vi "Durability_will_2012_07_05_long filesave working.vi"() -> ()   [LabVIEW 2011]
uses:
  <vilib>/DAQmx/write.llb/DAQmx Write (Counter Time 1Chan 1Samp).vi
  <vilib>/DAQmx/read.llb/DAQmx Read (Analog 1D Wfm NChan NSamp).vi
  <vilib>/express/express shared/ex_Modify Signal Name.vi
  <vilib>/measure/madcrms.llb/Basic Averaged DC-RMS for 1 Chan.vi
  <vilib>/DAQmx/miscellaneous.llb/DAQmx Fill In Error Info.vi
  <vilib>/express/express arith-compare/Formula/XNode/ExpressFormulaBlockNode.xnode
  <vilib>/measure/NI_MAPro.lvlib
  <vilib>/Analysis/NI_AALBase.lvlib
panel:
  out "Long":bool caption="Time has Elapsed"
  out "Short":bool caption="Time has Elapsed"
  out "Temps":dynamicdata(graph) caption="Signal Out"
  in  "View Short File":bool
  in  "View Long File":bool
  out "Power Graph":dynamicdata(graph) caption="Collected Signals"
  out "Errors":errorcluster
  out "RPM":dynamicdata(graph) caption="Collected Signals"
  in  "Long Filename":path=path "C:/Users/Will/Documents/LabVIEW Data/Durability/long.tdms" caption="Filename"
  in  "Short Filename":path=path "C:/Users/Will/Documents/LabVIEW Data/Durability/short.tdms" caption="Filename"
  out "Motor RPM":dbl format="%#.0f"
  out "Motor Power (watts)":dbl format="%#.4f"
  out "Power to MC1 (watts)":dbl format="%#.4f"
  out "Voltage to MC1 (volts)":dbl format="%#.4f"
  out "Current to MC1  (amps)":dbl format="%#.4f"
  in  "Manual Start":bool
  in  "Power \nSetting":i8(slide) min=0 max=100 step=10 scale=0.0..100.0
  out "Power Setting (%)":dbl format="%#.2f"
  out "Motor Temp (F)":dbl format="%.1f"
  out "Tank Temp (F)":dbl format="%.1f"
  in  "Quit 4":bool
  out "Motor Power Over Time":dbl(graph)
  out "Phase to Phase Voltage":waveform(dbl)(graph)
  out "Phase Current":waveform(dbl)(graph)
  # "Motor Power and RPM"
  # "Temperature"
  # "MC1"
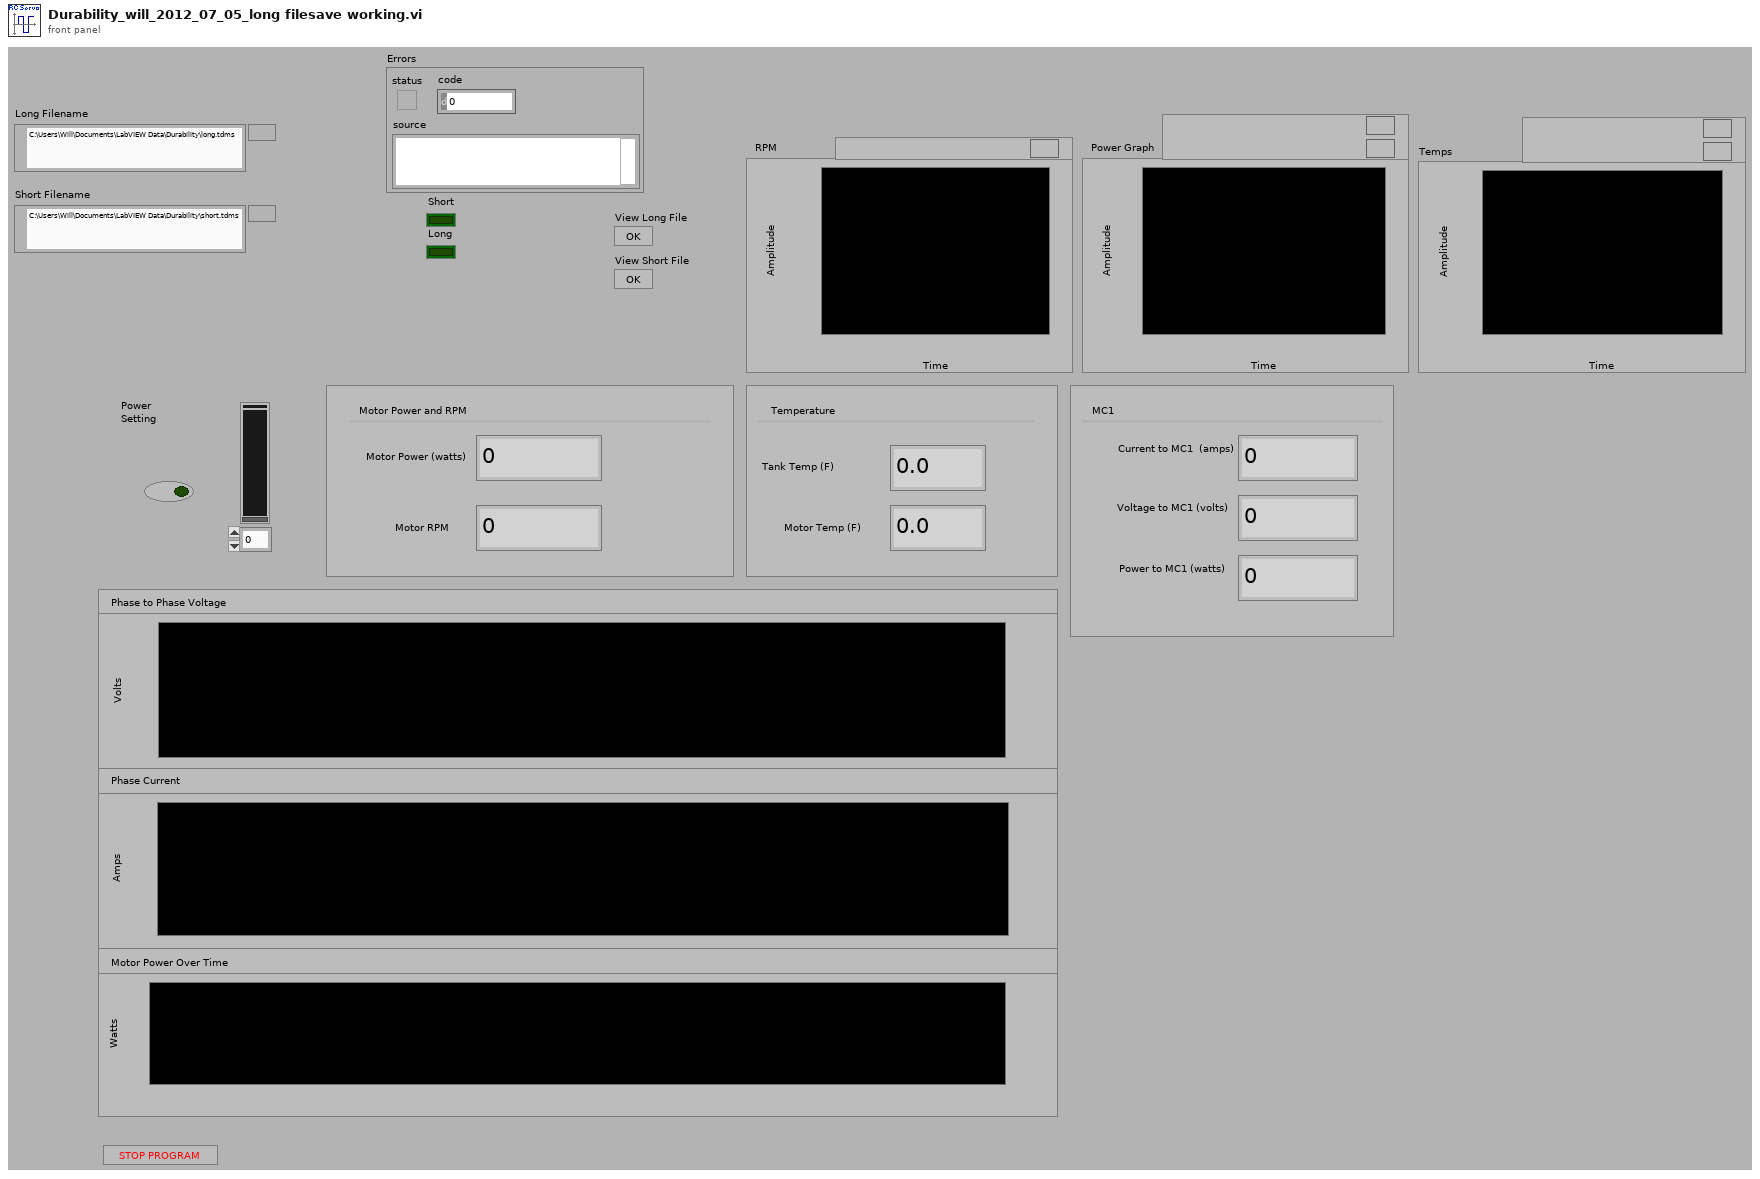
[diagram p1: front panel]
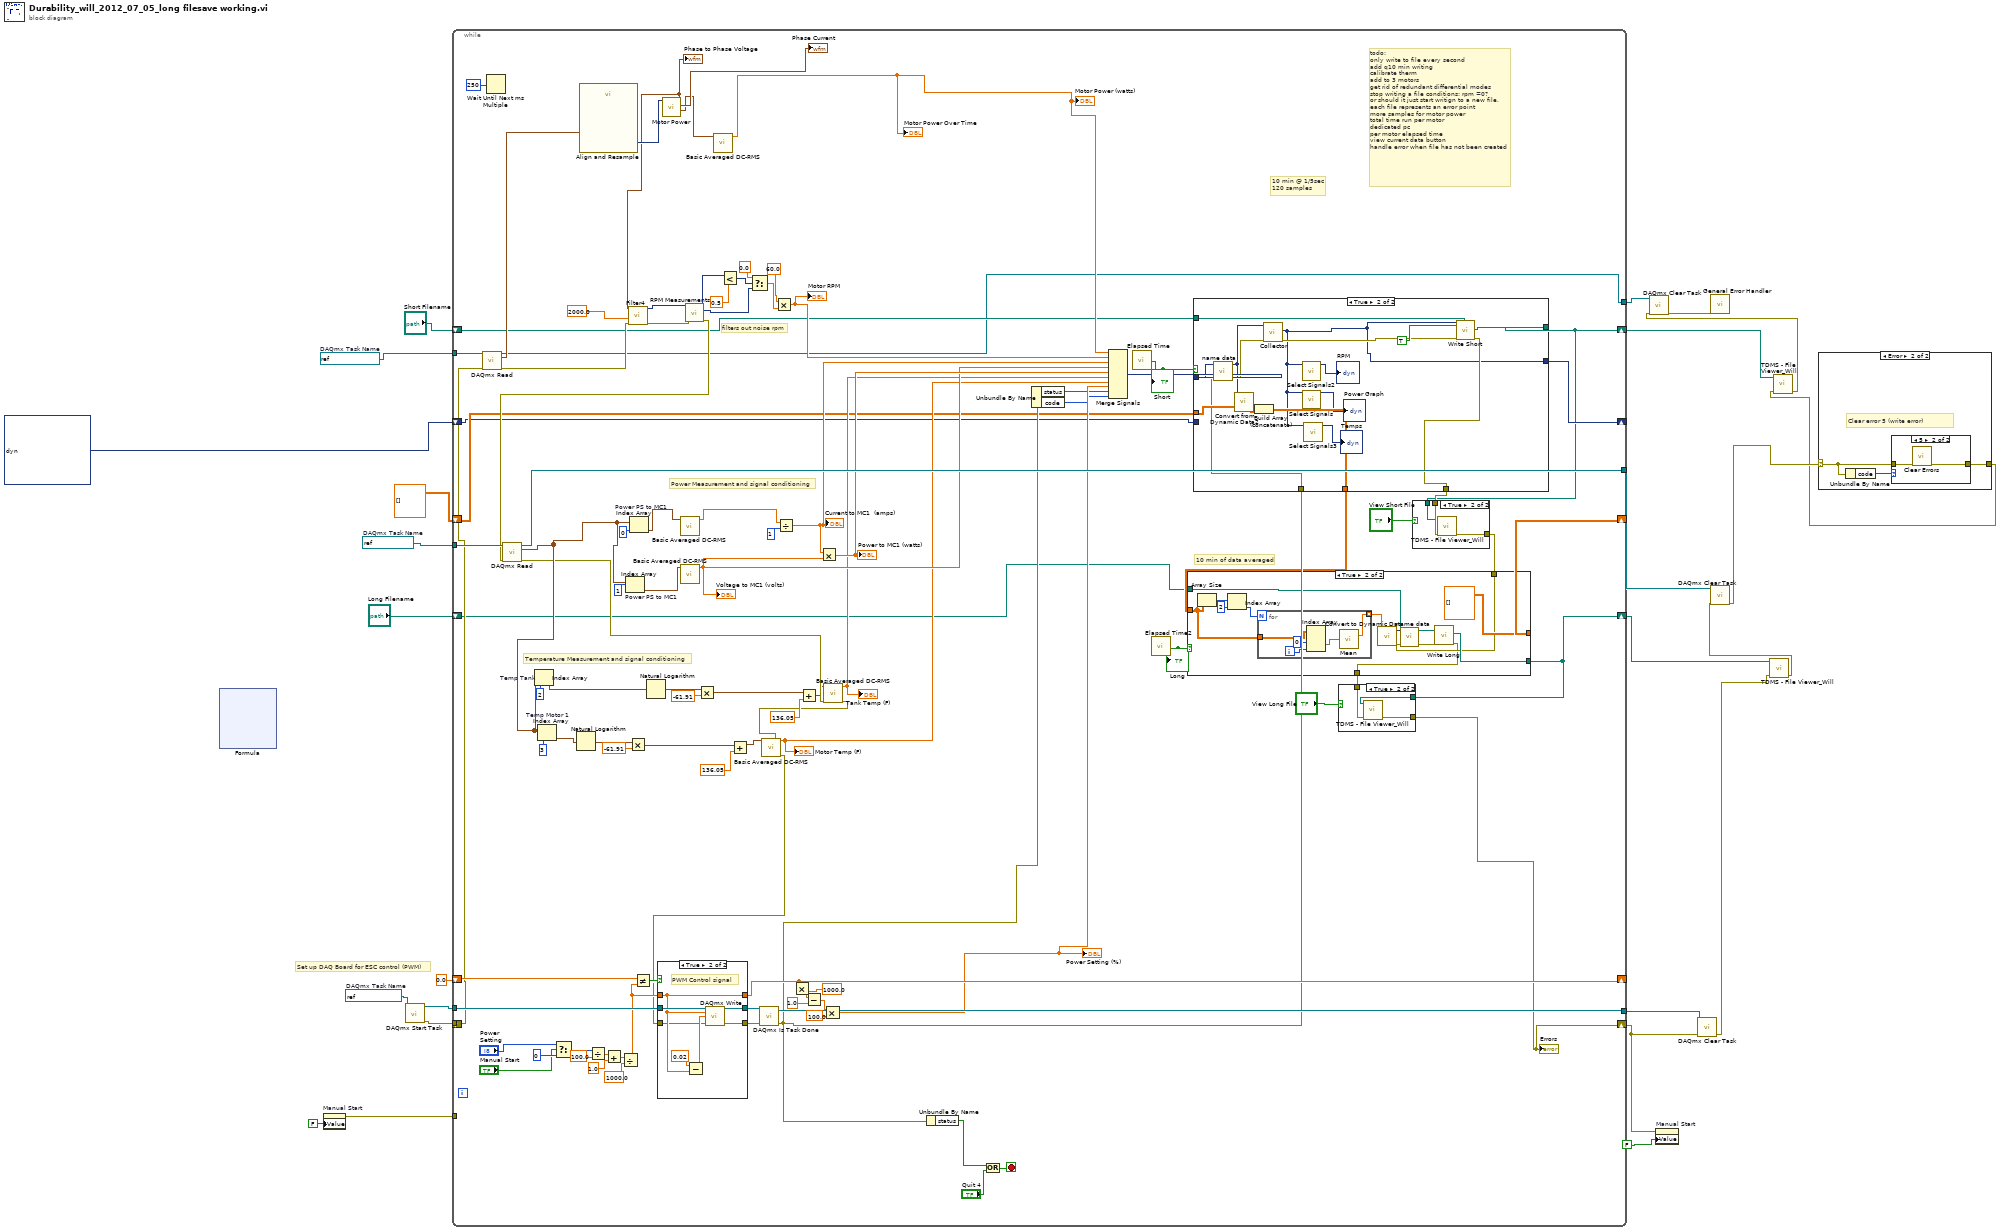
[diagram p0: block diagram]
diagram:
  w17 = refnum<k21> "PWM Signal"  # DAQmx Task Name
  w22 = refnum<k21> "MC Power"  # DAQmx Task Name
  w23 = refnum<k21> "Motor Power"  # DAQmx Task Name
  # "Set up DAQ Board for ESC control (PWM)"
  n1 = xnode "Formula"() -> ()  [unwired: 2 in, 2 out]
  n2 = property on="Manual Start" class="Bool (strict)"("Value"=FALSE ("Run Motor")) -> (error out=w20:errorcluster)  [unwired: 2 in, 1 out]
  n3 = call <vilib>:"DAQmx Start Task.vi"("task/channels in"=w17) -> ("task out"=w16:refnum<k21>, "error out"=w15:errorcluster)  [unwired: 13 in]
  n4 = while {
    tunnel: [w126] -> w25
    tunnel: w16 -> [w124]
    shift-right: [w107] -> _
    shift-left: 0.0 -> [w115]
    tunnel: w22 -> [w102]
    tunnel: [w101] -> w24
    tunnel: [w27] -> w5
    tunnel: w23 -> [w88]
    tunnel: w20 -> [_]
    tunnel: w15 -> [w81]
    shift-right: [w41] -> _
    shift-left: dbl[][][] [] -> [w40]
    shift-right: [w38] -> _
    shift-left: dynamicdata [{"t0"=timestamp(3424273593.297177 s since 1904-01-01), "dt"=1.0, "Y"=[0.36870916341083365, 0.42293065671747443, 0.3194538693360254, 0.34378340206924, 0.406287573514053, 5.427400356156832e-06, 5.564221456868835e-06], "attributes"=variant("NI_ChannelName"=variant(string "Collected"))}, {"t0"=timestamp(3424273593.297177 s since 1904-01-01), "dt"=1.0, "Y"=[36032.45951587244, 44745.94482180137, 36367.54666084641, 36357.44856318867, 45197.89735550279, 0.0, 0.0], "attributes"=variant("NI_ChannelName"=variant(string "Collected"))}, {"t0"=timestamp(3424273593.3551874 s since 1904-01-01), "dt"=1.0, "Y"=[0.1556021836894131, 0.15141620064378447, 0.1438458057740308, 0.1408303711788517, 0.14781549182338055, 0.055469397765108217, 0.05427340260921451], "attributes"=variant("NI_ChannelName"=variant(string "Collected"))}, {"t0"=timestamp(3424273593.3551874 s since 1904-01-01), "dt"=1.0, "Y"=[5.901053942994026, 5.9016644419685145, 5.9041573127810025, 5.904259062610079, 5.9029363148320275, 5.924914277913542, 5.925092340114435], "attributes"=variant("NI_ChannelName"=variant(string "Collected"))}, {"t0"=timestamp(3424273593.3551874 s since 1904-01-01), "dt"=1.0, "Y"=[0.9182168795988919, 0.8936076072773929, 0.8492882660736197, 0.8314989953234764, 0.8725454345789897, 0.3286514268057552, 0.32157492207180366], "attributes"=variant("NI_ChannelName"=variant(string "Collected"))}, {"t0"=timestamp(3424273593.3551874 s since 1904-01-01), "dt"=1.0, "Y"=[76.60774299226749, 76.60047605199273, 76.61680937553591, 76.62466019064554, 76.6657893466269, 76.66336109439426, 76.65005401148402], "attributes"=variant("NI_ChannelName"=variant(string "Collected"))}, {"t0"=timestamp(3424273593.3551874 s since 1904-01-01), "dt"=1.0, "Y"=[76.60066132165656, 76.60246802184979, 76.60186266099564, 76.60730576783594, 76.63755878876354, 76.62786739743993, 76.60729511945021], "attributes"=variant("NI_ChannelName"=variant(string "Collected"))}, {"t0"=timestamp(3424273593.37025 s since 1904-01-01), "dt"=1.0, "Y"=[39.99999999999999, 60.00000000000001, 30.000000000000004, 30.000000000000004, 80.0, 0.0, 0.0], "attributes"=variant("NI_ChannelName"=variant(string "Collected"))}, {"t0"=timestamp(3424273593.37025 s since 1904-01-01), "dt"=1.0, "Y"=[0.0, 0.0, 0.0, 0.0, 0.0, 0.0, 0.0], "attributes"=variant("NI_ChannelName"=variant(string "Collected"))}, {"t0"=timestamp(3424273593.37025 s since 1904-01-01), "dt"=1.0, "Y"=[20352.0, 20352.0, 20352.0, 20352.0, 20352.0, 20352.0, 20352.0], "attributes"=variant("NI_ChannelName"=variant(string "Collected"))}] ("Collected Signals 2") -> [w37]
    shift-right: [w28] -> w14
    shift-left: "Short Filename" -> [w36]
    shift-right: [w32] -> w8
    shift-left: "Long Filename" -> [w35]
    shift-right: [w26] -> w18
    shift-left: _ -> [_]
    stop <- w84 stop-if-true
    # "10 min of data averaged"
    # "todo:\nonly write to file every second\nadd q10 min writing\ncalibrate therm\nadd to 3 motors\nget rid of redundant differential modes\nstop writing a file conditions: rpm =0?\nor should it just start writign to a new file,\neach file represents an error point\nmore samples for motor power\ntotal time run per motor\ndedicated pc\nper motor elapsed time\nview current data button\nhandle error when file has not been created"
    # "filters out noise rpm"
    # "10 min @ 1/5sec\n120 samples"
    # "Power Measurement and signal conditioning"
    # "Temperature Measurement and signal conditioning"
    n5 = call-poly <vilib>:"DAQmx Read.vi"("task/channels in"=w88, "error in"=w81) -> ("task out"=w27:refnum<k21>, "data"=w63:waveform(dbl)[], "error out"=w98:errorcluster)  [unwired: 11 in]
    n6 = Wait Until Next ms Multiple(millisecond multiple=u32 250) -> ()  [unwired: 1 out]
    n7 = Select(t="Power \nSetting", s="Manual Start", f=i8 0) -> (s? t:f=w113:i8)
    n8 = call "Align and Resample"("Signals"=w63) -> ("Resampled Signals"=w64:dynamicdata)  [unwired: 8 in, 2 out]
    n9 = Divide(x=w113, y=100.0) -> (x/y=w119:dbl)
    n10 = Add(x=w119, y=1.0 ("x/y")) -> (x+y=w117:dbl)
    n11 = Divide(x=w117, y=1000.0) -> (x/y=w116:dbl)
    n12 = Not Equal?(x=w115, y=w116) -> (x != y?=w125:bool)
    n13 = call "Motor Power.vi"("data"=w64) -> ("Waveform"=w56:waveform(dbl), "Phase Current"=→"Phase Current":waveform(dbl), "Phase to Phase Voltage"=w61:waveform(dbl))  [unwired: 7 in, 1 out]
    "Phase to Phase Voltage" <- w61
    n14 = call "Filter4"("error in (no error)"=w98, "Lower Cut-Off"=2000.0 ("LowPass Filter CutOff [Hz]"), "Signal"=w61) -> ("error out"=w99:errorcluster, "Filtered Signal"=w90:dynamicdata)  [unwired: 7 in]
    n15 = call "RPM Measurements"("error in (no error)"=w99, "Signals"=w90) -> ("error out"=w83:errorcluster, "Frequency"=w94:dynamicdata, "Amplitude"=w91:dynamicdata)  [unwired: 7 in]
    n16 = call-poly <vilib>:"DAQmx Read.vi"("task/channels in"=w102, "error in"=w83) -> ("task out"=w101:refnum<k21>, "data"=w49:waveform(dbl)[], "error out"=w47:errorcluster)  [unwired: 11 in]
    n17 = Index Array "Temp Tank"(array=w49, index=2) -> (element=w50:waveform(dbl))
    n18 = Index Array "Temp Motor 1"(array=w49, index=3) -> (element=w76:waveform(dbl))
    n19 = Natural Logarithm(1:w76) -> (0:w80:waveform(dbl))
    n20 = Index Array "Power PS to MC1"(array=w49, index=1) -> (element=w52:waveform(dbl))
    n21 = Multiply(x=w80, y=-61.91) -> (x*y=w78:waveform(dbl))
    n22 = Index Array "Power PS to MC1"(array=w49, index=0) -> (element=w54:waveform(dbl))
    n23 = Natural Logarithm(1:w50) -> (0:w75:waveform(dbl))
    n24 = call-poly <vilib>:"Basic Averaged DC-RMS.vi"("signal in"=w54) -> ("DC value"=w53:dbl)  [unwired: 7 in, 3 out]
    n25 = call-poly <vilib>:"Basic Averaged DC-RMS.vi"("signal in"=w52) -> ("DC value"=w51:dbl)  [unwired: 7 in, 3 out]
    "Voltage to MC1 (volts)" <- w51
    n26 = Multiply(x=w75, y=-61.91) -> (x*y=w73:waveform(dbl))
    n27 = call-poly <vilib>:"Basic Averaged DC-RMS.vi"("signal in"=w56) -> ("DC value"=w55:dbl)  [unwired: 7 in, 3 out]
    "Motor Power Over Time" <- w55
    "Motor Power (watts)" <- w55
    n28 = Less?(x=w91, y=0.5) -> (x < y?=w93:dynamicdata)
    n29 = Add(x=w78, y=136.05) -> (x+y=w45:waveform(dbl))
    n30 = Select(t=0.0, s=w93, f=w94) -> (s? t:f=w96:dbl)
    n31 = Multiply(x=60.0, y=w96) -> (x*y=w70:dbl)
    "Motor RPM" <- w70
    n32 = Divide(x=w53, y=1) -> (x/y=w69:dbl)
    "Current to MC1  (amps)" <- w69
    n33 = Add(x=w73, y=136.05) -> (x+y=w46:waveform(dbl))
    n34 = Multiply(x=w69, y=w51) -> (x*y=w68:dbl)
    "Power to MC1 (watts)" <- w68
    n35 = call-poly <vilib>:"Basic Averaged DC-RMS.vi"("error in (no error)"=w47, "signal in"=w46) -> ("error out"=w42:errorcluster, "DC value"=w48:dbl)  [unwired: 6 in, 2 out]
    "Tank Temp (F)" <- w48
    n36 = call-poly <vilib>:"Basic Averaged DC-RMS.vi"("error in (no error)"=w42, "signal in"=w45) -> ("error out"=w43:errorcluster, "DC value"=w44:dbl)  [unwired: 6 in, 2 out]
    "Motor Temp (F)" <- w44
    n37 = case shown="True" w125 {
      tunnel: w116 -> [w177 w180]
      tunnel: w124 -> [w178 w184]
      tunnel: [w178 w182] -> w123
      tunnel: [w176 w181] -> w122
      tunnel: [w177 w180] -> w107
      tunnel: w43 -> [w176 w179]
      frame False {
      }
      frame True {
        # "PWM Control signal"
        n38 = Subtract(x=0.02, y=w180) -> (x-y=w183:dbl)
        n39 = call-poly <vilib>:"DAQmx Write.vi"("task/channels in"=w184, "high time"=w180, "low time"=w183, "error in"=w179) -> ("task out"=w182:refnum<k21>, "error out"=w181:errorcluster)  [unwired: 9 in, 1 out]
      }
    }
    n40 = call <vilib>:"DAQmx Is Task Done.vi"("task/channels in"=w123, "error in"=w122) -> ("task out"=w126:refnum<k21>, "error out"=w60:errorcluster)  [unwired: 11 in, 1 out]
    n41 = Multiply(x=w107, y=1000.0) -> (x*y=w108:dbl)
    n42 = Subtract(x=w108, y=1.0) -> (x-y=w111:dbl)
    n43 = Multiply(x=w111, y=100.0) -> (x*y=w67:dbl)
    "Power Setting (%)" <- w67
    n44 = Unbundle By Name(w60) -> ("status"=w82:bool)
    n45 = Or(x=w82, y="Quit 4") -> (x .or. y?=w84:bool)
    n46 = Unbundle By Name(w60) -> ("status"=w66:bool, "code"=w65:i32)
    n47 = Merge Signals(w55, w70, w69, w51, w68, w48, w44, w67, w66, w65) -> (w57:dynamicdata)
    n48 = call "Elapsed Time"() -> ("Time has Elapsed"=w59:bool)  [unwired: 12 in, 7 out]
    "Short" <- w59
    n49 = call "Elapsed Time2"() -> ("Time has Elapsed"=w58:bool)  [unwired: 12 in, 7 out]
    "Long" <- w58
    n50 = case shown="True" w59 {
      tunnel: w57 -> [_ w168]
      tunnel: w60 -> [w159 w165]
      tunnel: [w159 w161] -> w31
      tunnel: w36 -> [w158 w172]
      tunnel: [w158 w171] -> w28
      tunnel: [w157 w175] -> w39
      tunnel: w40 -> [w157 w174]
      tunnel: [w156 w160] -> w38
      tunnel: w37 -> [w156 _]
      frame False {
      }
      frame True {
        n51 = call "name data.vi"("error in (no error)"=w165, "Dynamic Data"=w168) -> ("error out"=w166:errorcluster, "Output"=w167:dynamicdata)  [unwired: 8 in]
        n52 = call "Convert from Dynamic Data2"("Dynamic Data Type"=w167) -> ("Array"=w173:dbl[][])  [unwired: 3 in]
        n53 = Build Array (concatenate)(w174, w173) -> (w175:dbl[][][])
        n54 = call "Collector"("error in (no error)"=w166, "Signals"=w167) -> ("error out"=w162:errorcluster, "Collected Signals"=w160:dynamicdata)  [unwired: 8 in]
        n55 = call "Select Signals2"("Signals"=w160) -> ("Signal Out"=→"RPM":dynamicdata)  [unwired: 9 in, 1 out]
        n56 = call "Select Signals"("Signals"=w160) -> ("Signal Out"=→"Power Graph":dynamicdata)  [unwired: 9 in, 1 out]
        n57 = call "Select Signals3"("Signals"=w160) -> ("Signal Out"=→"Temps":dynamicdata)  [unwired: 9 in, 1 out]
        n58 = call "Write Short"("Signals"=w160, "Reset"=TRUE, "error in (no error)"=w162, "Filename"=w172) -> ("Filename Out"=w171:path, "error out"=w161:errorcluster)  [unwired: 13 in, 1 out]
      }
    }
    n59 = case shown="True" "View Short File" {
      tunnel: w31 -> [w127 w130]
      tunnel: [w127 w129] -> w30
      tunnel: w28 -> [_ w128]
      frame False {
      }
      frame True {
        n60 = call "TDMS - File Viewer_Will.vi"("error in (no error)"=w130, "file path"=w128) -> ("error out"=w129:errorcluster)  [unwired: 5 out]
      }
    }
    n61 = case shown="True" w58 {
      tunnel: w39 -> [w136 w148]
      tunnel: [w137 w150] -> w32
      tunnel: w35 -> [w137 w149]
      tunnel: [w136 dbl[][][] []] -> w41
      tunnel: w30 -> [w135 w140]
      tunnel: [w135 w138] -> w29
      frame False {
      }
      frame True {
        n62 = Array Size(array=w148) -> (size(s)=w144:i32[])
        n63 = Index Array(array=w144, index=2) -> (element=w145:i32)
        n64 = for {
          N: w145 -> [_]
          tunnel: w148 -> [w155]
          tunnel: [w151] -> w143 mode=indexing
          i -> [w154]
          n65 = Index Array(array=w155, index (dim 1)=0 ("disabled index (row)"), index (dim 2)=w154) -> (element=w153:dbl[])  [unwired: 1 in]
          n66 = call <vilib>:"Mean.vi"("X"=w153) -> ("mean"=w151:dbl)  [unwired: 1 out]
        }
        n67 = call "Convert to Dynamic Data"("Array"=w143) -> ("Dynamic Data Type"=w142:dynamicdata)  [unwired: 3 in]
        n68 = call "name data.vi"("error in (no error)"=w140, "Dynamic Data"=w142) -> ("error out"=w139:errorcluster, "Output"=w141:dynamicdata)  [unwired: 8 in]
        n69 = call "Write Long"("Signals"=w141, "error in (no error)"=w139, "Filename"=w149) -> ("Filename Out"=w150:path, "error out"=w138:errorcluster)  [unwired: 14 in, 1 out]
      }
    }
    n70 = case shown="True" "View Long File" {
      tunnel: w32 -> [_ w134]
      tunnel: w29 -> [w131 w133]
      tunnel: [w131 w132] -> w26
      frame False {
      }
      frame True {
        n71 = call "TDMS - File Viewer_Will.vi"("error in (no error)"=w133, "file path"=w134) -> ("error out"=w132:errorcluster)  [unwired: 5 out]
      }
    }
    "Errors" <- w26
  }
  n72 = property on="Manual Start" class="Bool (strict)"(error in=w18, "Value"=FALSE ("Run Motor")) -> ()  [unwired: 1 in, 2 out]
  n73 = call <vilib>:"DAQmx Clear Task.vi"("task in"=w25, "error in"=w18) -> ("error out"=w7:errorcluster)  [unwired: 13 in]
  n74 = call "TDMS - File Viewer_Will.vi"("error in (no error)"=w7, "file path"=w8) -> ("error out"=w6:errorcluster)  [unwired: 5 out]
  n75 = call <vilib>:"DAQmx Clear Task.vi"("task in"=w24, "error in"=w6) -> ("error out"=w2:errorcluster)  [unwired: 13 in]
  n76 = case shown="Error" w2 {
    selector: w2 -> [w186 w188]
    tunnel: [w186 w187] -> w1
    frame No Error {
    }
    frame Error {
      # "Clear error 5 (write error)"
      n77 = Unbundle By Name(w188) -> ("code"=w189:i32)
      n78 = case shown="5" w189 {
        tunnel: w188 -> [w190 w192]
        tunnel: [w190 w191] -> w187
        frame Default {
        }
        frame 5 {
          n79 = call <vilib>:"Clear Errors.vi"("error in (no error)"=w192) -> ("error out"=w191:errorcluster)  [unwired: 6 in]
        }
      }
    }
  }
  n80 = call "TDMS - File Viewer_Will.vi"("error in (no error)"=w1, "file path"=w14) -> ("error out"=w3:errorcluster)  [unwired: 5 out]
  n81 = call <vilib>:"DAQmx Clear Task.vi"("task in"=w5, "error in"=w3) -> ("error out"=w4:errorcluster)  [unwired: 13 in]
  n82 = call <vilib>:"General Error Handler.vi"("error in (no error)"=w4) -> ()  [unwired: 10 in, 5 out]
